vi "LinearSystem_CalculateX.vi"(8 "dT_Seconds":dbl, 9 "ClampedU":T1, 10 "X":T1, 11 "Linearsystem":T2) -> (0 "Error":bool, 3 "X":T1)   [LabVIEW 2019, in "Trajectory_Library.lvlib"]
doc: "Creates a new LINEAR SYSTEM data cluster with the specified values. \n\n\nInputs: \n - XXX -- XXX.\n\nOutputs:\n - XXX -- XXX."
uses:
  Trajectory_Library.lvlib
  LINEAR_SYSTEM.ctl
  <vilib>/Analysis/Matrix/Datatypes/RealMatrix.ctl
  <vilib>/Analysis/baseanly.llb/Real A x B.vi
  <vilib>/Analysis/7linalg.llb/Matrix Exp.vi
  <vilib>/Analysis/7linalg.llb/Real Matrix Exp.vi
  <vilib>/Analysis/Matrix/Numeric/Multiply/Multiply.vi
  <vilib>/Analysis/Matrix/Numeric/Multiply/Multiply - RM,R.vi
  <vilib>/Analysis/Matrix/Numeric/Add/Add - RM,RM.vi
  <vilib>/Analysis/NI_AALBase.lvlib
  <vilib>/Analysis/Matrix/NI_Matrix.lvlib
panel:
  # "<States,States>"
  # "<States,Inputs>"
  # "<Outputs,States>"
  # "<Outputs,Inputs>"
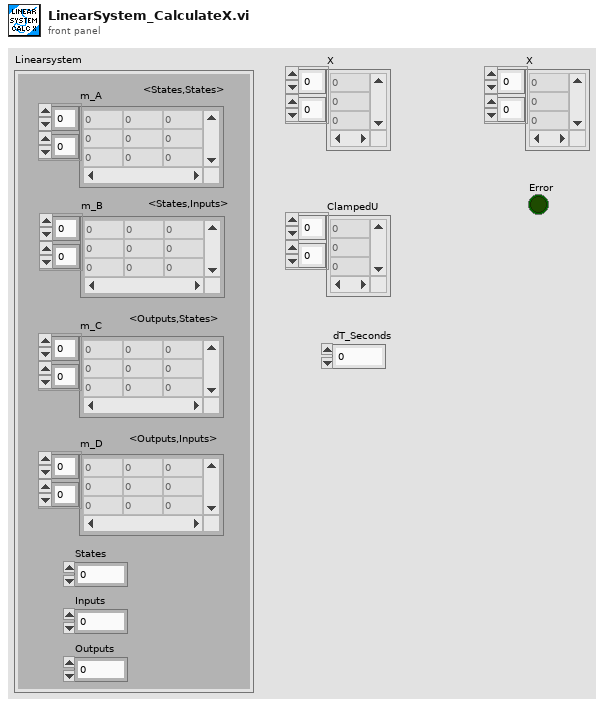
[diagram p1: front panel]
types:
  T1 = typedef "NI_Matrix.lvlib/RealMatrix.ctl" = dbl[][]
  T2 = typedef "Trajectory_Library.lvlib/LINEAR_SYSTEM.ctl" = cluster{"m_A":T1, "m_B":T1, "m_C":T1, "m_D":T1, "States":i32, "Inputs":i32, "Outputs":i32}
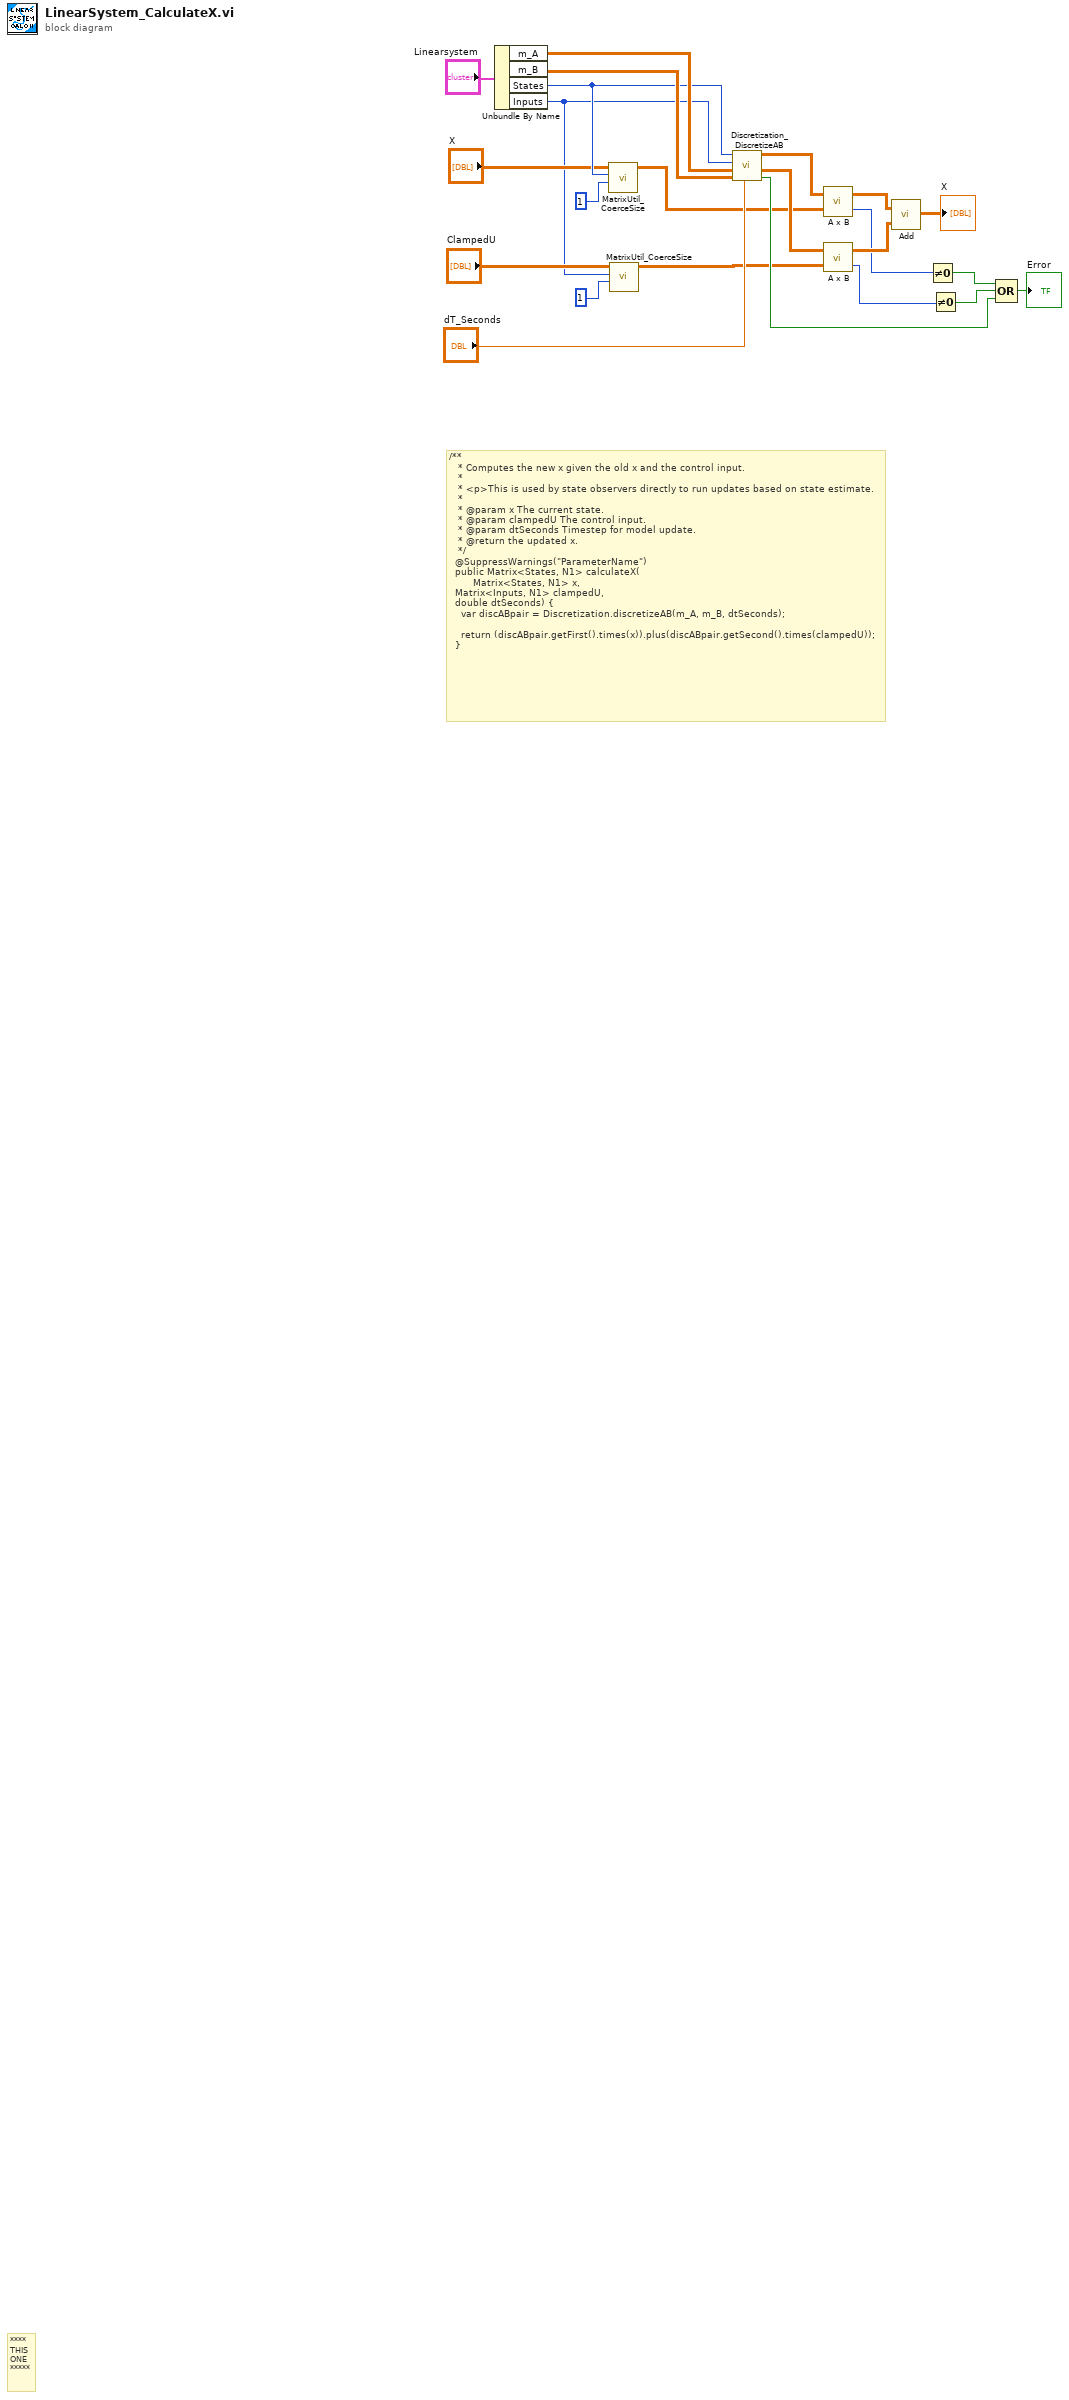
[diagram p0: block diagram]
diagram:
  # "/**\n   * Computes the new x given the old x and the control input.\n   *\n   * <p>This is used by state observers directly to run updates based on state estimate.\n   *\n   * @param x The current state.\n   * @param clampedU The control input.\n   * @param dtSeconds Timestep for model update.\n   * @return the updated x.\n   */\n  @SuppressWarnings(\"ParameterName\")\n  public Matrix<States, N1> calculateX(\n      \t\tMatrix<States, N1> x, \n\t\tMatrix<Inputs, N1> clampedU, \n\t\tdouble dtSeconds) {\n    var discABpair = Discretization.discretizeAB(m_A, m_B, dtSeconds);\n\n    return (discABpair.getFirst().times(x)).plus(discABpair.getSecond().times(clampedU));\n  }"
  # "****\nTHIS\nONE\n*****"
  n1 = Unbundle By Name("Linearsystem") -> ("m_A"=w22:T1, "m_B"=w21:T1, "States"=w8:i32, "Inputs"=w3:i32)
  n2 = call "MatrixUtil_CoerceSize.vi"("Columns"=1 ("number of columns"), "Rows"=w8, "input matrix"="X") -> ("output matrix"=w5:T1)  [unwired: 8 in]
  n3 = call "MatrixUtil_CoerceSize.vi"("Columns"=1 ("number of columns"), "Rows"=w3, "input matrix"="ClampedU") -> ("output matrix"=w1:T1)  [unwired: 8 in]
  n4 = call "Discretization_DiscretizeAB.vi"("dT_Seconds"="dT_Seconds", "ContB"=w21, "ContA"=w22, "Inputs"=w3, "States"=w8) -> ("Error"=w12:bool, "DiscB"=w18:T1, "DiscA"=w19:T1)  [unwired: 4 in]
  n5 = call-poly <vilib>:"A x B.vi"("B"=w5, "A"=w19) -> ("error"=w10:i32, "A x B"=w17:T1)
  n6 = call-poly <vilib>:"A x B.vi"("B"=w1, "A"=w18) -> ("error"=w11:i32, "A x B"=w16:T1)
  n7 = call-poly <vilib>:"Add.vi"("Real Matrix B"=w16, "Real Matrix A"=w17) -> ("A + B"=→"X":T1)
  n8 = Not Equal To 0?(x=w10) -> (x != 0?=w14:bool)
  n9 = Not Equal To 0?(x=w11) -> (x != 0?=w13:bool)
  n10 = Compound Arithmetic op=OR(w14, w13, w12) -> (→"Error":bool)
